vi "OE2052_DATA Transmit.vi"(0 "Input Data":u8[](array[numeric])) -> (1 "Parameter Values":T2, 2 "Total Data Array":dbl[][](array[numeric]), 3 "A&B_PLL&Overload":T1)   [LabVIEW 2011]
panel:
  out "B_Overload":u8
  out "B_PLL":u8
  out "A_Overload":u8
  out "A_PLL":u8
  out "A_X":dbl[](array[numeric])
  out "A_Y":dbl[](array[numeric])
  out "A_R":dbl[](array[numeric])
  out "A_Xita":dbl[](array[numeric])
  out "B_X":dbl[](array[numeric])
  out "B_Y":dbl[](array[numeric])
  out "B_R":dbl[](array[numeric])
  out "B_Xita":dbl[](array[numeric])
  out "B_Freq":dbl[](array[numeric])
  out "A_Freq":dbl[](array[numeric])
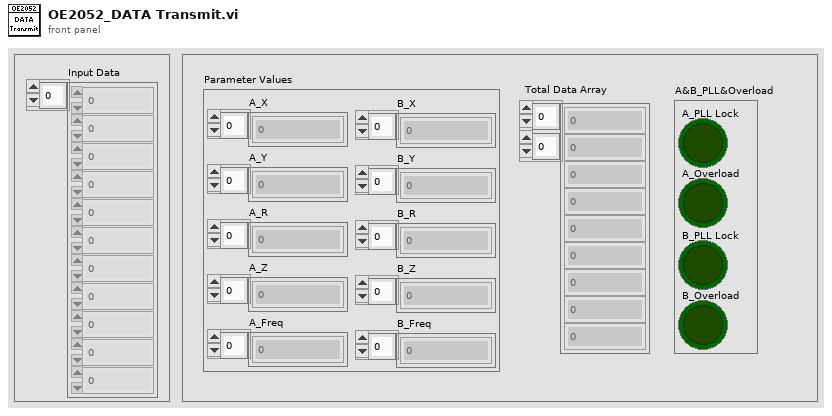
[diagram p1: front panel]
types:
  T1 = cluster{"A_PLL Lock":bool, "A_Overload":bool, "B_PLL Lock":bool, "B_Overload":bool}
  T2 = cluster{"A_X":dbl[], "A_Y":dbl[], "A_R":dbl[], "A_Z":dbl[], "A_Freq":dbl[], "B_X":dbl[], "B_Y":dbl[], "B_R":dbl[], "B_Z":dbl[], "B_Freq":dbl[]}
  T3 = cluster{"A_X":dbl[], "A_Y":dbl[], "A_R":dbl[], "A_Xita":dbl[], "A_Freq":dbl[], "B_X":dbl[], "B_Y":dbl[], "B_R":dbl[], "B_Xita":dbl[], "B_Freq":dbl[]}
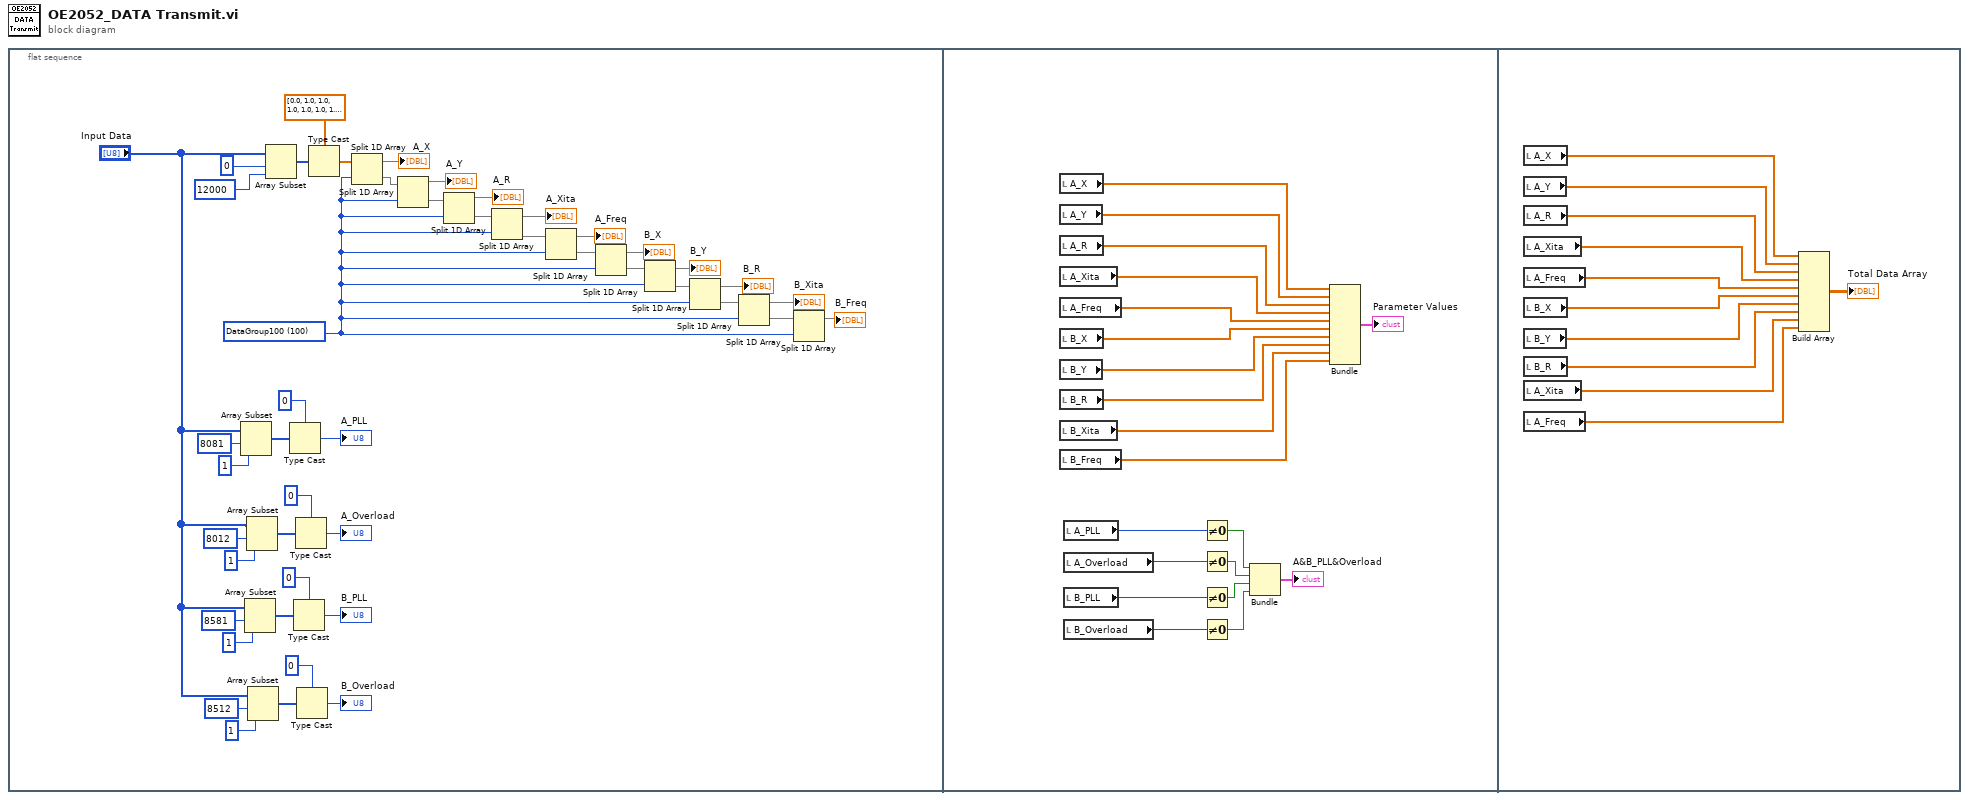
[diagram p0: block diagram]
diagram:
  n1 = flat-sequence {
    frame #0 {
      w22 = u16 100 items=["unsignedInt8"=1, "unsignedInt16"=2, "unsignedInt32"=4, "unsignedInt64"=8, "Float"=80, "Double"=160, "StartLength"=2240, "DataGroup50"=50, "DataGroup100"=100, "DataGroup20"=20] ("数据类型")
      n2 = Array Subset(array="Input Data", index=8081 ("索引"), length=1 ("长度")) -> (w19:u8[])
      n3 = Array Subset(array="Input Data", index=8581 ("索引"), length=1 ("长度")) -> (w9:u8[])
      n4 = Array Subset(array="Input Data", index=8012 ("索引"), length=1 ("长度")) -> (w14:u8[])
      n5 = Array Subset(array="Input Data", index=8512 ("索引"), length=1 ("长度")) -> (w4:u8[])
      n6 = Array Subset(array="Input Data", index=0 ("索引"), length=12000 ("长度")) -> (w43:u8[])
      n7 = Type Cast(type=u8 0, x=w19) -> (*(type *) &x=→"A_PLL":u8)
      n8 = Type Cast(type=u8 0, x=w9) -> (*(type *) &x=→"B_PLL":u8)
      n9 = Type Cast(type=u8 0, x=w14) -> (*(type *) &x=→"A_Overload":u8)
      n10 = Type Cast(type=u8 0, x=w4) -> (*(type *) &x=→"B_Overload":u8)
      n11 = Type Cast(type=dbl[] [0.0, 1.0, 1.0, 1.0, 1.0, 1.0, 1.0, 1.0, 1.0, 1.0, 1.0, 1.0, 1.0, 1.0, 1.0, 1.0, 1.0, 1.0, 1.0, 1.0, 1.0, 1.0, 1.0, 1.0, 1.0, 1.0, 1.0, 1.0, 1.0, 1.0, 1.0, 1.0, 1.0, 1.0, 1.0, 1.0, 1.0, 1.0, 1.0, 1.0, 1.0, 1.0, 1.0, 1.0, 1.0, 1.0, 1.0, 1.0, 1.0, 1.0, 1.0, 1.0, 1.0, 1.0, 1.0, 1.0, 1.0, 1.0, 1.0, 1.0, 1.0, 1.0, 1.0, 1.0, 1.0, 1.0, 1.0, 1.0, 1.0, 1.0, 1.0, 1.0, 1.0, 1.0, 1.0, 1.0, 1.0, 1.0, 1.0, 1.0, 1.0, 1.0, 1.0, 1.0, 1.0, 1.0, 1.0, 1.0, 1.0, 1.0, 1.0, 1.0, 1.0, 1.0, 1.0, 1.0, 1.0, 1.0, 1.0, 1.0, 1.0, 1.0, 1.0, 1.0, 1.0, 1.0, 1.0, 1.0, 1.0, 1.0, 1.0, 1.0, 1.0, 1.0, 1.0, 1.0, 1.0, 1.0, 1.0, 1.0, 1.0, 1.0, 1.0, 1.0, 1.0, 1.0, 1.0, 1.0, 1.0, 1.0, 1.0, 1.0, 1.0, 1.0, 1.0, 1.0, 1.0, 1.0, 1.0, 1.0, 1.0, 1.0, 1.0, 1.0, 1.0, 1.0, 1.0, 1.0, 1.0, 1.0, 1.0, 1.0, 1.0, 1.0, 1.0, 1.0, 1.0, 1.0, 1.0, 1.0, 1.0, 1.0, 1.0, 1.0, 1.0, 1.0, 1.0, 1.0, 1.0, 1.0, 1.0, 1.0, 1.0, 1.0, 1.0, 1.0, 1.0, 1.0, 1.0, 1.0, 1.0, 1.0, 1.0, 1.0, 1.0, 1.0, 1.0, 1.0, 1.0, 1.0, 1.0, 1.0, 1.0, 1.0, 1.0, 1.0, 1.0, 1.0, 1.0, 1.0, 1.0, 1.0, 1.0, 1.0, 1.0, 1.0, 1.0, 1.0, 1.0, 1.0, 1.0, 1.0, 1.0, 1.0, 1.0, 1.0, 1.0, 1.0, 1.0, 1.0, 1.0, 1.0, 1.0, 1.0, 1.0, 1.0, 1.0, 1.0, 1.0, 1.0, 1.0, 1.0, 1.0, 1.0, 1.0, 1.0, 1.0, 1.0, 1.0, 1.0, 1.0, 1.0, 1.0, 1.0, 1.0, 1.0, 1.0, 1.0, 1.0, 1.0, 1.0, 1.0, 1.0, 1.0, 1.0, 1.0, 1.0, 1.0, 1.0, 1.0, 1.0, 1.0, 1.0, 1.0, 1.0, 1.0, 1.0, 1.0, 1.0, 1.0, 1.0, 1.0, 1.0, 1.0, 1.0, 1.0, 1.0, 1.0, 1.0, 1.0, 1.0, 1.0, 1.0, 1.0, 1.0, 1.0, 1.0, 1.0, 1.0, 1.0, 1.0, 1.0, 1.0, 1.0, 1.0, 1.0, 1.0, 1.0, 1.0, 1.0, 1.0, 1.0, 1.0, 1.0, 1.0, 1.0, 1.0, 1.0, 1.0, 1.0, 1.0, 1.0, 1.0, 1.0, 1.0, 1.0, 1.0, 1.0, 1.0, 1.0, 1.0, 1.0, 1.0, 1.0, 1.0, 1.0, 1.0, 1.0, 1.0, 1.0, 1.0, 1.0, 1.0, 1.0, 1.0, 1.0, 1.0, 1.0, 1.0, 1.0, 1.0, 1.0, 1.0, 1.0, 1.0, 1.0, 1.0, 1.0, 1.0, 1.0, 1.0, 1.0, 1.0, 1.0, 1.0, 1.0, 1.0, 1.0, 1.0, 1.0, 1.0, 1.0, 1.0, 1.0, 1.0, 1.0, 1.0, 1.0, 1.0, 1.0, 1.0, 1.0, 1.0, 1.0, 1.0, 1.0, 1.0, 1.0, 1.0, 1.0, 1.0, 1.0, 1.0, 1.0, 1.0, 1.0, 1.0, 1.0, 1.0, 1.0, 1.0, 1.0, 1.0, 1.0, 1.0, 1.0, 1.0, 1.0, 1.0, 1.0, 0.0, 1.0, 1.0, 1.0, 1.0, 1.0, 1.0, 1.0, 1.0, 1.0, 1.0, 1.0, 1.0, 1.0, 1.0, 1.0, 1.0, 1.0, 1.0, 1.0, 1.0, 1.0, 1.0, 1.0, 1.0, 1.0, 1.0, 1.0, 1.0, 1.0, 1.0, 1.0, 1.0, 1.0, 1.0, 1.0, 1.0, 1.0, 1.0, 1.0, 1.0, 1.0, 1.0, 1.0, 1.0, 1.0, 1.0, 1.0, 1.0, 1.0, 1.0, 1.0, 1.0, 1.0, 1.0, 1.0, 1.0, 1.0, 1.0, 1.0, 1.0, 1.0, 1.0, 1.0, 1.0, 1.0, 1.0, 1.0, 1.0, 1.0, 1.0, 1.0, 1.0, 1.0, 1.0, 1.0, 1.0, 1.0, 1.0, 1.0, 1.0, 1.0, 1.0, 1.0, 1.0, 1.0, 1.0, 1.0, 1.0, 1.0, 1.0, 1.0, 1.0, 1.0, 1.0, 1.0, 1.0, 1.0, 1.0, 1.0, 1.0, 1.0, 1.0, 1.0, 1.0, 1.0, 1.0, 1.0, 1.0, 1.0, 1.0, 1.0, 1.0, 1.0, 1.0, 1.0, 1.0, 1.0, 1.0, 1.0, 1.0, 1.0, 1.0, 1.0, 1.0, 1.0, 1.0, 1.0, 1.0, 1.0, 1.0, 1.0, 1.0, 1.0, 1.0, 1.0, 1.0, 1.0, 1.0, 1.0, 1.0, 1.0, 1.0, 1.0, 1.0, 1.0, 1.0, 1.0, 1.0, 1.0, 1.0, 1.0, 1.0, 1.0, 1.0, 1.0, 1.0, 1.0, 1.0, 1.0, 1.0, 1.0, 1.0, 1.0, 1.0, 1.0, 1.0, 1.0, 1.0, 1.0, 1.0, 1.0, 1.0, 1.0, 1.0, 1.0, 1.0, 1.0, 1.0, 1.0, 1.0, 1.0, 1.0, 1.0, 1.0, 1.0, 1.0, 1.0, 1.0, 1.0, 1.0, 1.0, 1.0, 1.0, 1.0, 1.0, 1.0, 1.0, 1.0, 1.0, 1.0, 1.0, 1.0, 1.0, 1.0, 1.0, 1.0, 1.0, 1.0, 1.0, 1.0, 1.0, 1.0, 1.0, 1.0, 1.0, 1.0, 1.0, 1.0, 1.0, 1.0, 1.0, 1.0, 1.0, 1.0, 1.0, 1.0, 1.0, 1.0, 1.0, 1.0, 1.0, 1.0, 1.0, 1.0, 1.0, 1.0, 1.0, 1.0, 1.0, 1.0, 1.0, 1.0, 1.0, 1.0, 1.0, 1.0, 1.0, 1.0, 1.0, 1.0, 1.0, 1.0, 1.0, 1.0, 1.0, 1.0, 1.0, 1.0, 1.0, 1.0, 1.0, 1.0, 1.0, 1.0, 1.0, 1.0, 1.0, 1.0, 1.0, 1.0, 1.0, 1.0, 1.0, 1.0, 1.0, 1.0, 1.0, 1.0, 1.0, 1.0, 1.0, 1.0, 1.0, 1.0, 1.0, 1.0, 1.0, 1.0, 1.0, 1.0, 1.0, 1.0, 1.0, 1.0, 1.0, 1.0, 1.0, 1.0, 1.0, 1.0, 1.0, 1.0, 1.0, 1.0, 1.0, 1.0, 1.0, 1.0, 1.0, 1.0, 1.0, 1.0, 1.0, 1.0, 1.0, 1.0, 1.0, 1.0, 1.0, 1.0, 1.0, 1.0, 1.0, 1.0, 1.0, 1.0, 1.0, 1.0, 1.0, 1.0, 1.0, 1.0, 1.0, 1.0, 1.0, 1.0, 1.0, 1.0, 1.0, 1.0, 1.0, 1.0, 1.0, 1.0, 1.0, 1.0, 1.0, 1.0, 1.0, 1.0, 1.0, 1.0, 1.0, 1.0, 1.0, 1.0, 1.0, 1.0, 1.0, 1.0, 1.0, 1.0, 1.0, 1.0, 1.0, 1.0, 1.0, 1.0, 1.0, 1.0, 1.0, 1.0, 1.0, 1.0, 1.0, 1.0, 1.0, 1.0, 1.0, 1.0, 1.0, 1.0, 1.0, 1.0, 1.0, 1.0, 1.0, 1.0, 1.0, 1.0, 1.0, 1.0, 1.0, 1.0, 1.0, 1.0, 1.0, 1.0, 1.0], x=w43) -> (*(type *) &x=w38:dbl[])
      n12 = Split 1D Array(array=w38, index=w22) -> (first subarray=→"A_X":dbl[], second subarray=w39:dbl[])
      n13 = Split 1D Array(array=w39, index=w22) -> (first subarray=→"A_Y":dbl[], second subarray=w44:dbl[])
      n14 = Split 1D Array(array=w44, index=w22) -> (first subarray=→"A_R":dbl[], second subarray=w31:dbl[])
      n15 = Split 1D Array(array=w31, index=w22) -> (first subarray=→"A_Xita":dbl[], second subarray=w33:dbl[])
      n16 = Split 1D Array(array=w33, index=w22) -> (first subarray=→"A_Freq":dbl[], second subarray=w32:dbl[])
      n17 = Split 1D Array(array=w32, index=w22) -> (first subarray=→"B_X":dbl[], second subarray=w42:dbl[])
      n18 = Split 1D Array(array=w42, index=w22) -> (first subarray=→"B_Y":dbl[], second subarray=w45:dbl[])
      n19 = Split 1D Array(array=w45, index=w22) -> (first subarray=→"B_R":dbl[], second subarray=w46:dbl[])
      n20 = Split 1D Array(array=w46, index=w22) -> (first subarray=→"B_Xita":dbl[], second subarray=w35:dbl[])
      n21 = Split 1D Array(array=w35, index=w22) -> (first subarray=→"B_Freq":dbl[])  [unwired: 1 out]
    }
    frame #1 {
      n22 = local read "A_X"() -> (w66:dbl[])
      n23 = local read "A_Y"() -> (w65:dbl[])
      n24 = local read "A_R"() -> (w64:dbl[])
      n25 = local read "A_Xita"() -> (w63:dbl[])
      n26 = local read "A_Freq"() -> (w62:dbl[])
      n27 = local read "B_X"() -> (w61:dbl[])
      n28 = local read "B_Y"() -> (w60:dbl[])
      n29 = local read "B_R"() -> (w59:dbl[])
      n30 = local read "B_Xita"() -> (w58:dbl[])
      n31 = local read "B_Freq"() -> (w57:dbl[])
      n32 = local read "A_PLL"() -> (w49:u8)
      n33 = local read "A_Overload"() -> (w50:u8)
      n34 = local read "B_PLL"() -> (w51:u8)
      n35 = local read "B_Overload"() -> (w52:u8)
      n36 = Not Equal To 0?(x=w49) -> (x != 0?=w54:bool)
      n37 = Not Equal To 0?(x=w50) -> (x != 0?=w55:bool)
      n38 = Not Equal To 0?(x=w51) -> (x != 0?=w53:bool)
      n39 = Not Equal To 0?(x=w52) -> (x != 0?=w48:bool)
      n40 = Bundle(w54, w55, w53, w48) -> (→"A&B_PLL&Overload":cluster{bool, bool, bool, bool})  [unwired: 1 in]
      n41 = Bundle("A_X"=w66, "A_Y"=w65, "A_R"=w64, "A_Xita"=w63, "A_Freq"=w62, "B_X"=w61, "B_Y"=w60, "B_R"=w59, "B_Xita"=w58, "B_Freq"=w57) -> (→"Parameter Values":T3)  [unwired: 1 in]
    }
    frame #2 {
      n42 = local read "A_X"() -> (w70:dbl[])
      n43 = local read "A_Y"() -> (w71:dbl[])
      n44 = local read "A_R"() -> (w72:dbl[])
      n45 = local read "A_Xita"() -> (w73:dbl[])
      n46 = local read "A_Freq"() -> (w74:dbl[])
      n47 = local read "B_X"() -> (w75:dbl[])
      n48 = local read "B_Y"() -> (w76:dbl[])
      n49 = local read "B_R"() -> (w77:dbl[])
      n50 = local read "A_Xita"() -> (w67:dbl[])
      n51 = local read "A_Freq"() -> (w68:dbl[])
      n52 = Build Array(w70, w71, w72, w73, w74, w75, w76, w77, w67, w68) -> (→"Total Data Array":dbl[][])
    }
  }
